vi "control number color.vi"(8 "arrivée traitement":string[][](array[string])) -> (0 "nb orange":dbl, 1 "nb blue":dbl, 2 "nb yellow":dbl, 3 "nb white":dbl, 4 "nb green":dbl, 5 "nb red":dbl, 6 "True":bool, 7 "False":bool)   [LabVIEW 2019]
uses:
  <vilib>/regexp/Match Regular Expression.xnode
panel:
  out "RubixTab patron 2":string[][](array[string])
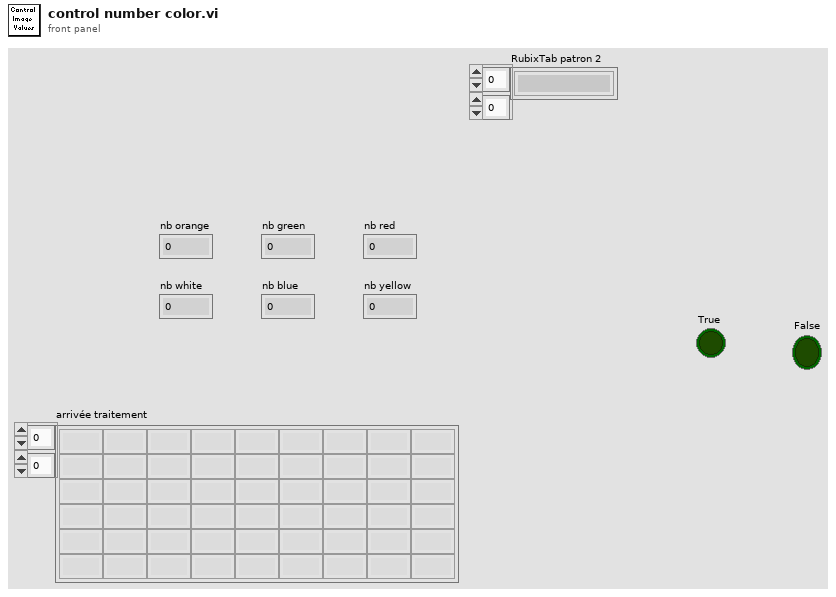
[diagram p1: front panel]
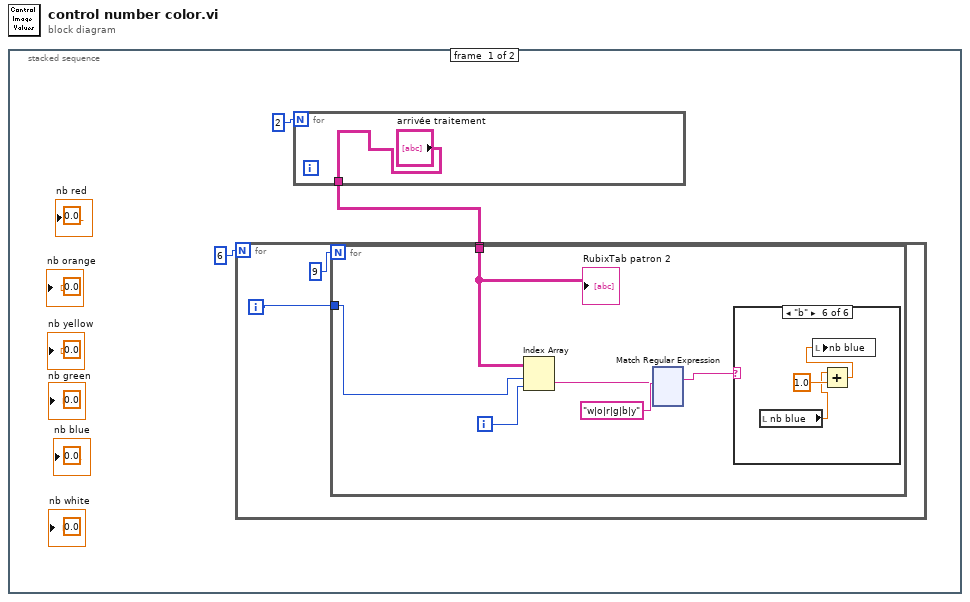
[diagram p0: block diagram]
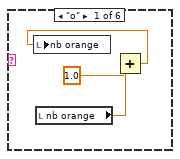
[diagram p2: hidden frame]
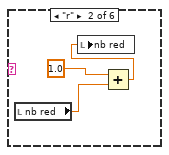
[diagram p3: hidden frame]
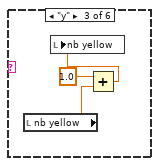
[diagram p4: hidden frame]
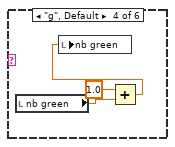
[diagram p5: hidden frame]
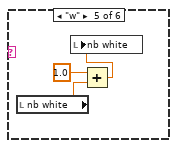
[diagram p6: hidden frame]
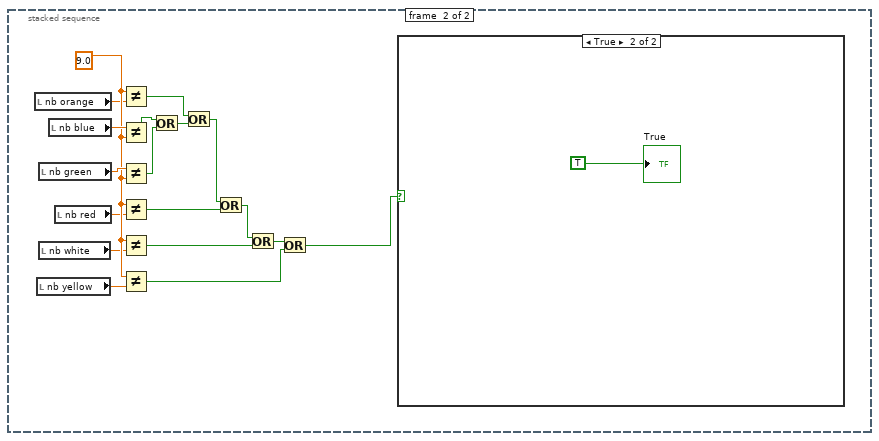
[diagram p7: hidden frame]
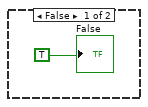
[diagram p8: hidden frame]
diagram:
  n1 = stacked-sequence {
    frame #0 {
      n2 = for {
        N: 2 -> [_]
        tunnel: ["arrivée traitement"] -> w8
      }
      n3 = for {
        N: 6 -> [_]
        tunnel: w8 -> [w11]
        i -> [w13]
        n4 = for {
          N: 9 -> [_]
          tunnel: w13 -> [w18]
          tunnel: w11 -> [w19]
          i -> [w17]
          n5 = Index Array(array=w19, index (row)=w18, index (col)=w17) -> (element=w15:string)
          n6 = xnode "Match Regular Expression"("input string"=w15, "regular expression"="w|o|r|g|b|y" ("input string")) -> ("whole match"=w14:string)  [unwired: 4 in, 4 out]
          n7 = case shown="\"b\"" w14 {
            frame "o" {
              n8 = local read "nb orange"() -> (w136:dbl)
              n9 = Add(x=1.0, y=w136) -> (x+y=w134:dbl)
              n10 = local write "nb orange"(w134) -> ()
            }
            frame "r" {
              n11 = local read "nb red"() -> (w138:dbl)
              n12 = Add(x=1.0, y=w138) -> (x+y=w137:dbl)
              n13 = local write "nb red"(w137) -> ()
            }
            frame "y" {
              n14 = local read "nb yellow"() -> (w142:dbl)
              n15 = Add(x=1.0, y=w142) -> (x+y=w141:dbl)
              n16 = local write "nb yellow"(w141) -> ()
            }
            frame "g", Default {
              n17 = local read "nb green"() -> (w145:dbl)
              n18 = Add(x=1.0, y=w145) -> (x+y=w144:dbl)
              n19 = local write "nb green"(w144) -> ()
            }
            frame "w" {
              n20 = local read "nb white"() -> (w147:dbl)
              n21 = Add(x=1.0, y=w147) -> (x+y=w148:dbl)
              n22 = local write "nb white"(w148) -> ()
            }
            frame "b" {
              n23 = local read "nb blue"() -> (w149:dbl)
              n24 = Add(x=w149, y=1.0) -> (x+y=w150:dbl)
              n25 = local write "nb blue"(w150) -> ()
            }
          }
          "RubixTab patron 2" <- w19
        }
      }
      "nb red" <- 0.0
      "nb orange" <- 0.0
      "nb yellow" <- 0.0
      "nb green" <- 0.0
      "nb blue" <- 0.0
      "nb white" <- 0.0
    }
    frame #1 {
      w165 = 9.0 ("y")
      n26 = local read "nb orange"() -> (w162:dbl)
      n27 = local read "nb yellow"() -> (w161:dbl)
      n28 = local read "nb green"() -> (w168:dbl)
      n29 = local read "nb white"() -> (w164:dbl)
      n30 = local read "nb blue"() -> (w169:dbl)
      n31 = local read "nb red"() -> (w163:dbl)
      n32 = Not Equal?(x=w165, y=w162) -> (x != y?=w160:bool)
      n33 = Not Equal?(x=w169, y=w165) -> (x != y?=w167:bool)
      n34 = Not Equal?(x=w168, y=w165) -> (x != y?=w166:bool)
      n35 = Not Equal?(x=w165, y=w163) -> (x != y?=w157:bool)
      n36 = Not Equal?(x=w165, y=w164) -> (x != y?=w155:bool)
      n37 = Not Equal?(x=w165, y=w161) -> (x != y?=w153:bool)
      n38 = Or(x=w167, y=w166) -> (x .or. y?=w159:bool)
      n39 = Or(x=w160, y=w159) -> (x .or. y?=w158:bool)
      n40 = Or(x=w158, y=w157) -> (x .or. y?=w156:bool)
      n41 = Or(x=w156, y=w155) -> (x .or. y?=w154:bool)
      n42 = Or(x=w154, y=w153) -> (x .or. y?=w152:bool)
      n43 = case shown="True" w152 {
        frame False {
          "False" <- TRUE
        }
        frame True {
          "True" <- TRUE
        }
      }
    }
  }
